vi "Sort Tree Items by Numerical order.vi"(6 "Reverse Order?":bool, 8 "error in":errorcluster, 9 "Sort Column":i32, 10 "Tag (\"\")":string, 11 "Data Tree":refnum<vi>) -> (0 "error out":errorcluster)   [LabVIEW 2010]
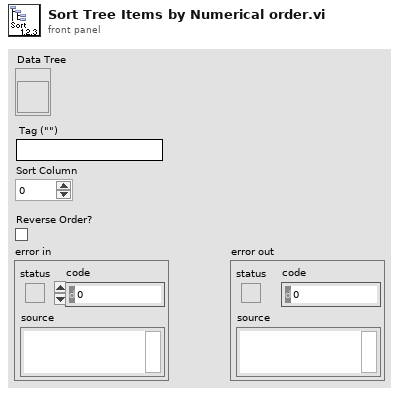
[diagram p1: front panel]
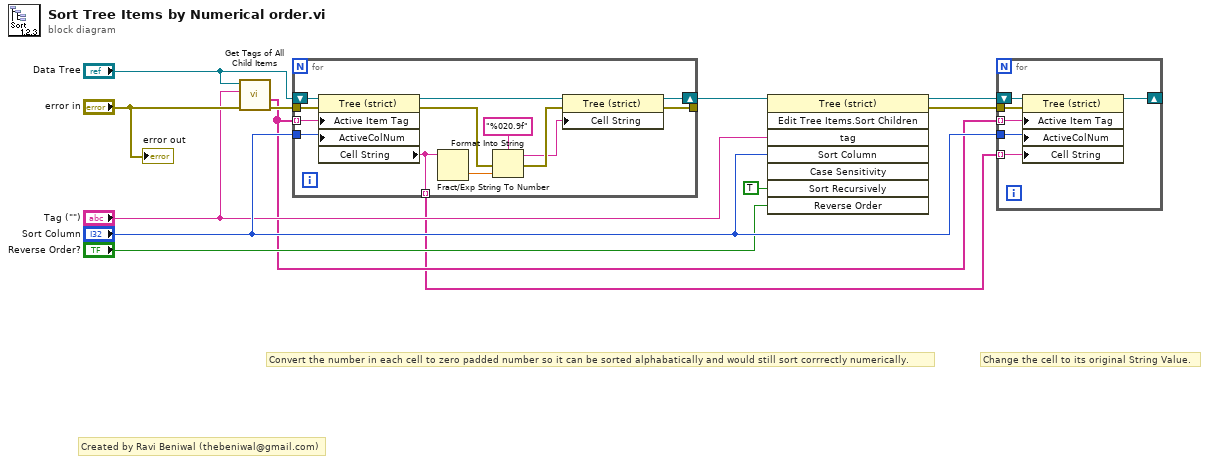
[diagram p0: block diagram]
diagram:
  # "Change the cell to its original String Value."
  # "Convert the number in each cell to zero padded number so it can be sorted alphabatically and would still sort corrrectly numerically."
  # "Created by Ravi Beniwal (thebeniwal@gmail.com)"
  n1 = call "Get Tags of All Child Items.vi"("error in"="error in", "Parent Tag"="Tag (\"\")", "Tree Ref in"="Data Tree") -> ("error out"=w7:errorcluster, "Tags of All Child Items"=w2:string[])  [unwired: 4 in, 3 out]
  n2 = for {
    shift-right: [w20] -> w5
    shift-left: "Data Tree" -> [w25]
    tunnel: w2 -> [w22] mode=indexing
    tunnel: w7 -> [w24]
    tunnel: "Sort Column" -> [w23]
    tunnel: [w19] -> _
    tunnel: [w14] -> w1 mode=indexing
    n3 = property class="Tree (strict)"(reference=w25, error in=w24, "Active Item Tag"=w22, "ActiveColNum"=w23) -> (reference out=w21:refnum<vi>, error out=w16:errorcluster, "Cell String"=w14:string)
    n4 = Fract/Exp String To Number(string=w14) -> (number=w17:dbl)  [unwired: 3 in, 1 out]
    n5 = Format Into String(format string="%020.9f", error in=w16, w17) -> (resulting string=w13:string, error out=w15:errorcluster)  [unwired: 1 in]
    n6 = property class="Tree (strict)"(reference=w21, error in=w15, "Cell String"=w13) -> (reference out=w20:refnum<vi>, error out=w19:errorcluster)
  }
  n7 = invoke on="Invoke Node" class="Tree (strict)" method="Edit Tree Items.Sort Children"(reference=w5, "tag"="Tag (\"\")", "Sort Column"="Sort Column", "Sort Recursively"=TRUE ("Sort Recursively?"), "Reverse Order"="Reverse Order?") -> (reference out=w4:refnum<vi>, error out=w3:errorcluster)  [unwired: 3 in, 6 out]
  n8 = for {
    shift-right: [w27] -> _
    shift-left: w4 -> [w31]
    tunnel: w2 -> [w28] mode=indexing
    tunnel: w3 -> [w30]
    tunnel: "Sort Column" -> [w29]
    tunnel: w1 -> [w26] mode=indexing
    n9 = property class="Tree (strict)"(reference=w31, error in=w30, "Active Item Tag"=w28, "ActiveColNum"=w29, "Cell String"=w26) -> (reference out=w27:refnum<vi>)  [unwired: 1 out]
  }
  "error out" <- "error in"
